vi "Ring to String.vi"(1 "Ring Ctrl Ref":refnum<vi>) -> (0 "Output String":string)   [LabVIEW 2023, in "Utilities.lvlib"]
uses:
  Utilities.lvlib
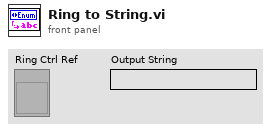
[diagram p1: front panel]
types:
  T1 = typedef "LVStringsAndValuesArrayTypeDef_U16.ctl" = cluster{"String":string, "Value":u16}[]
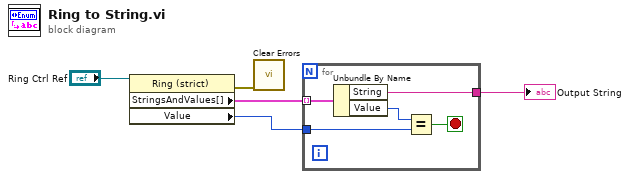
[diagram p0: block diagram]
diagram:
  n1 = property class="Ring (strict)"(reference="Ring Ctrl Ref") -> (error out=w2:errorcluster, "StringsAndValues[]"=w4:T1, "Value"=w3:u16)  [unwired: 1 in, 1 out]
  n2 = call <vilib>:"Clear Errors.vi"("error in (no error)"=w2) -> ()  [unwired: 5 in, 2 out]
  n3 = for {
    tunnel: w4 -> [w10] mode=indexing
    tunnel: w3 -> [w7]
    tunnel: [w9] -> w1
    stop <- w6 stop-if-true
    n4 = Unbundle By Name(w10) -> ("String"=w9:string, "Value"=w8:u16)
    n5 = Equal?(x=w8, y=w7) -> (x = y?=w6:bool)
  }
  "Output String" <- w1
